vi "Initiate.vi"(0 "VISA resource name":refnum<visa-resource-name>, 7 "Enable Continuous Initiation (False)":bool, 11 "error in (no error)":errorcluster) -> (4 "VISA resource name out":refnum<visa-resource-name>, 15 "error out":errorcluster)   [LabVIEW 2020, in "Keithley 27XX.lvlib"]
doc: "This VI sends the Initiate command to the instrument. It is used to begin scans and initiate measurements."
uses:
  Keithley 27XX.lvlib
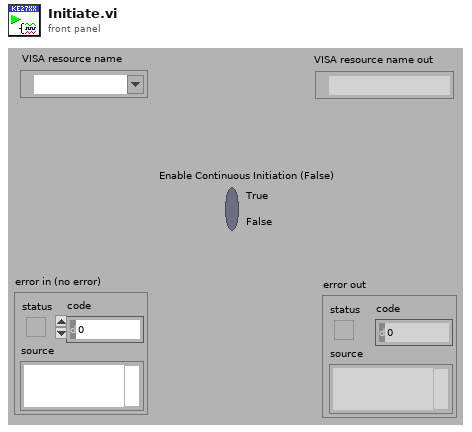
[diagram p1: front panel]
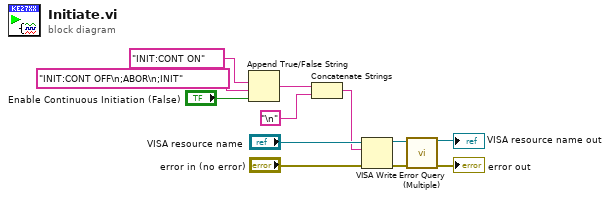
[diagram p0: block diagram]
diagram:
  n1 = Append True/False String(1:"Enable Continuous Initiation (False)", 2:"INIT:CONT OFF\n;ABOR\n;INIT" ("write buffer"), 3:"INIT:CONT ON" ("true string")) -> (0:w2:string)  [unwired: 1 in]
  n2 = Concatenate Strings(w2, "\n") -> (w1:string)
  n3 = VISA Write(VISA resource name="VISA resource name", write buffer=w1, error in (no error)="error in (no error)") -> (VISA resource name out=w10:refnum<visa-resource-name>, error out=w9:errorcluster)  [unwired: 1 out]
  n4 = call "Error Query (Multiple).vi"("VISA resource name"=w10, "error in (no error)"=w9) -> ("VISA resource name out"=→"VISA resource name out":refnum<visa-resource-name>, "error out"=→"error out":errorcluster)  [unwired: 10 in, 2 out]
